vi "Select Replacement Terminal.vi"(10 "Terms[]":refnum<vi>[](array[refnum]), 11 "Terminal in":refnum<vi>) -> (3 "Terminal out":refnum<vi>)   [LabVIEW 2020, in "Message Maker.lvlib"]
uses:
  Message Maker.lvlib
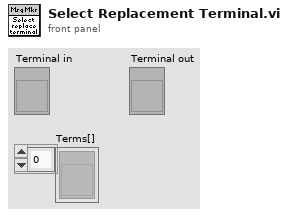
[diagram p1: front panel]
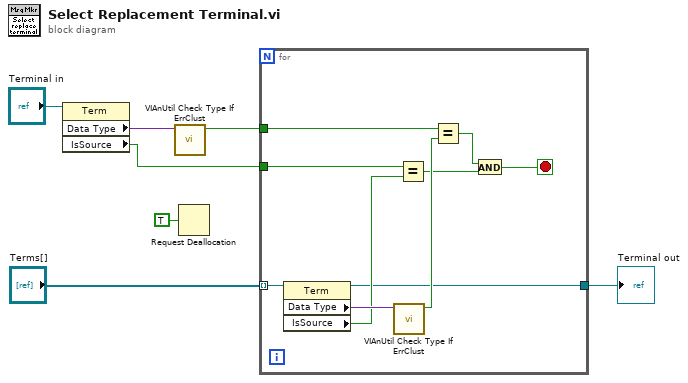
[diagram p0: block diagram]
diagram:
  n1 = property class="Term"(reference="Terminal in") -> ("Data Type"=w6:variant, "IsSource"=w4:bool)  [unwired: 1 in, 2 out]
  n2 = call <vilib>:"VIAnUtil Check Type If ErrClust.vi"("Data In"=w6) -> ("IsErrClust?"=w3:bool)  [unwired: 9 in, 1 out]
  n3 = Request Deallocation(TRUE ("flag")) -> ()
  n4 = for {
    tunnel: "Terms[]" -> [w16] mode=indexing
    tunnel: w4 -> [w15]
    tunnel: w3 -> [w13]
    tunnel: [w8] -> w2
    stop <- w9 stop-if-true
    n5 = property class="Term"(reference=w16) -> (reference out=w8:refnum<vi>, "Data Type"=w17:variant, "IsSource"=w14:bool)  [unwired: 1 in, 1 out]
    n6 = call <vilib>:"VIAnUtil Check Type If ErrClust.vi"("Data In"=w17) -> ("IsErrClust?"=w12:bool)  [unwired: 9 in, 1 out]
    n7 = Equal?(x=w15, y=w14) -> (x = y?=w10:bool)
    n8 = Equal?(x=w13, y=w12) -> (x = y?=w11:bool)
    n9 = And(x=w11, y=w10) -> (x .and. y?=w9:bool)
  }
  "Terminal out" <- w2
